vi "GetOVLError.vi"(8 "error in":errorcluster, 9 "rules":T1(array[cluster]), 10 "ctrl refs":cluster{"Ref":refnum<vi>, "value type":string}[](array[cluster]), 11 "status in (low: False, high: True, medium: not changed)":bool[](array[boolean])) -> (0 "error out":errorcluster, 1 "msg to email":string, 2 "Alarm? array":bool[](array[boolean]), 3 "status out (low: False, high: True, medium: not changed)":bool[](array[boolean]), 5 "values":dbl[](array[numeric]))   [LabVIEW 2017]
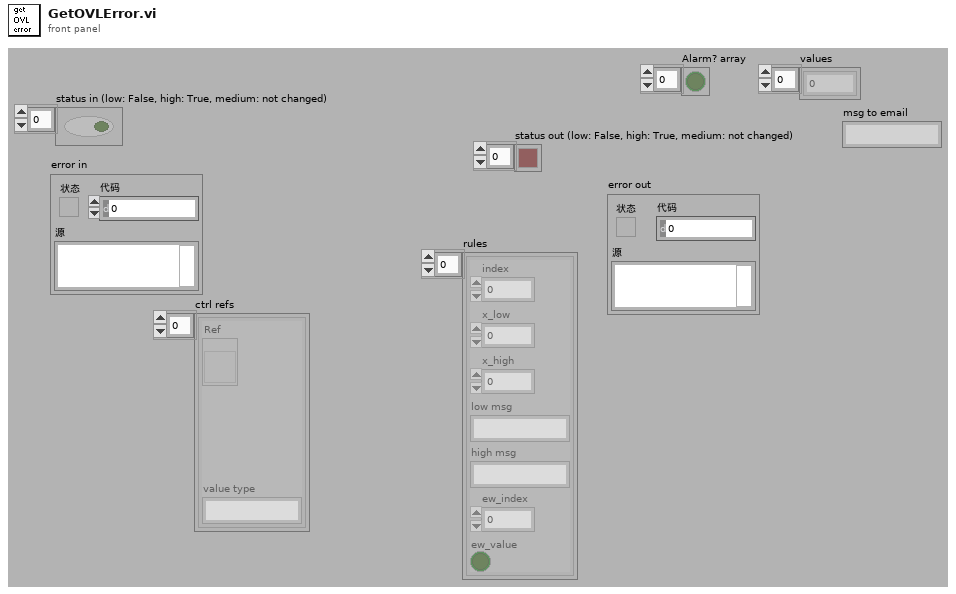
[diagram p1: front panel]
types:
  T1 = cluster{"index":i32, "x_low":dbl, "x_high":dbl, "low msg":string, "high msg":string, "ew_index":i32, "ew_value":bool}[]
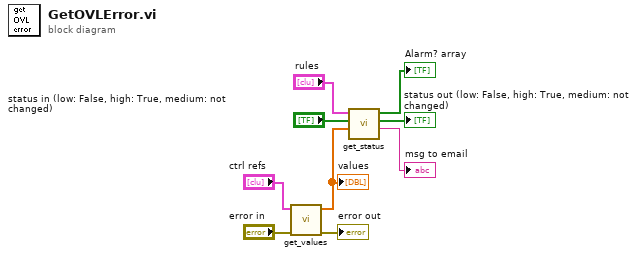
[diagram p0: block diagram]
diagram:
  n1 = call "get_values.vi"("error in"="error in", "ctrl refs"="ctrl refs") -> ("error out"=→"error out":errorcluster, "values"=w2:dbl[])  [unwired: 6 out]
  "values" <- w2
  n2 = call "get_status.vi"("values"=w2, "status in (low: False, high: True, medium: not changed)"="status in (low: False, high: True, medium: not changed)", "rules"="rules") -> ("msg to email"=→"msg to email":string, "status out (low: False, high: True, medium: not changed)"=→"status out (low: False, high: True, medium: not changed)":bool[], "Alarms? array"=→"Alarm? array":bool[])  [unwired: 4 out]
